vi "Write Register (Core).vi"(0 "SLSC Local in":refnum<class "SLSC Local.lvclass">, 1 "type":enum16{"U8", "U16", "U32", "U64"}(ring), 5 "device":refnum<k21>="$DefaultDevices", 7 "register address":u32 format="%.0x", 9 "data":u64 format="%.0x", 11 "error in (no error)":errorcluster) -> (4 "SLSC Local out":refnum<class "SLSC Local.lvclass">, 6 "device out":refnum<k21>, 8 "next register address":u32 format="%.0x", 15 "error out":errorcluster)   [LabVIEW 2015, in "SLSC Interfaces.lvlib" / "SLSC Local.lvclass"]
uses:
  SLSC Local.lvclass
  <vilib>/SLSC/Write Register (U64).vi
  <vilib>/SLSC/Write Register (U32).vi
  <vilib>/SLSC/Write Register (U16).vi
  <vilib>/SLSC/Write Register (U8).vi
  <vilib>/SLSC/SLSC.lvlib
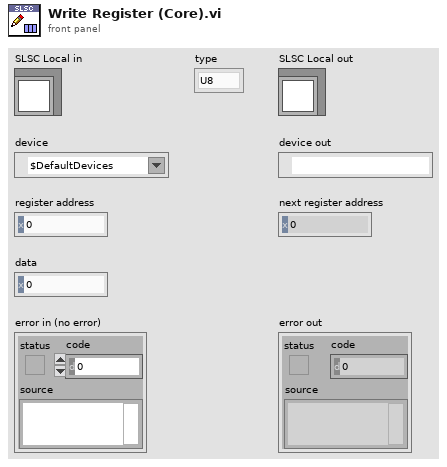
[diagram p1: front panel]
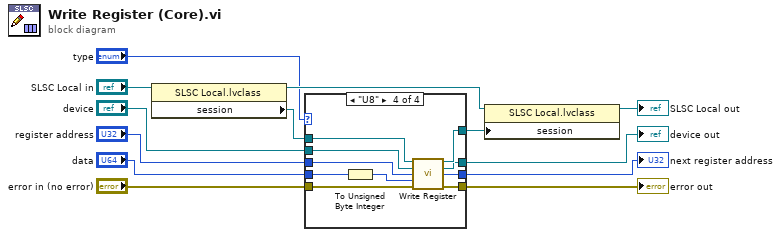
[diagram p0: block diagram]
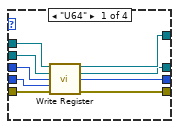
[diagram p2: hidden frame]
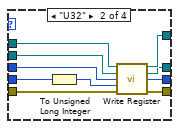
[diagram p3: hidden frame]
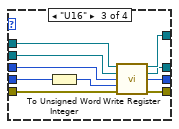
[diagram p4: hidden frame]
diagram:
  n1 = property class="SLSC Local.lvclass"(reference="SLSC Local in") -> (reference out=w6:refnum<class "SLSC Local.lvclass">, "session"=w5:refnum<k21>)  [unwired: 1 in, 1 out]
  n2 = case shown="\"U8\"" "type" {
    tunnel: [w22 w32 w42 w52] -> w13
    tunnel: [w21 w31 w41 w51] -> w12
    tunnel: "error in (no error)" -> [w20 w30 w40 w50]
    tunnel: "data" -> [w19 w24 w34 w44]
    tunnel: "register address" -> [w18 w29 w39 w49]
    tunnel: "device" -> [w17 w28 w38 w48]
    tunnel: w5 -> [w16 w27 w37 w47]
    tunnel: [w15 w26 w36 w46] -> w4
    tunnel: [w14 w25 w35 w45] -> w3
    frame "U64" {
      n3 = call-poly <vilib>:"Write Register.vi"("session in"=w16, "device"=w17, "register address"=w18, "data"=w19, "error in (no error)"=w20) -> ("session out"=w15:refnum<k21>, "device out"=w14:refnum<k21>, "next register address"=w22:u32, "error out"=w21:errorcluster)  [unwired: 7 in]
    }
    frame "U32" {
      n4 = To Unsigned Long Integer(number=w24) -> (unsigned 32bit integer=w23:u32)
      n5 = call-poly <vilib>:"Write Register.vi"("session in"=w27, "device"=w28, "register address"=w29, "data"=w23, "error in (no error)"=w30) -> ("session out"=w26:refnum<k21>, "device out"=w25:refnum<k21>, "next register address"=w32:u32, "error out"=w31:errorcluster)  [unwired: 7 in]
    }
    frame "U16" {
      n6 = To Unsigned Word Integer(number=w34) -> (unsigned 16bit integer=w33:u16)
      n7 = call-poly <vilib>:"Write Register.vi"("session in"=w37, "device"=w38, "register address"=w39, "data"=w33, "error in (no error)"=w40) -> ("session out"=w36:refnum<k21>, "device out"=w35:refnum<k21>, "next register address"=w42:u32, "error out"=w41:errorcluster)  [unwired: 7 in]
    }
    frame "U8" {
      n8 = To Unsigned Byte Integer(number=w44) -> (unsigned 8bit integer=w43:u8)
      n9 = call-poly <vilib>:"Write Register.vi"("session in"=w47, "device"=w48, "register address"=w49, "data"=w43, "error in (no error)"=w50) -> ("session out"=w46:refnum<k21>, "device out"=w45:refnum<k21>, "next register address"=w52:u32, "error out"=w51:errorcluster)  [unwired: 7 in]
    }
  }
  "error out" <- w12
  "device out" <- w3
  "next register address" <- w13
  n10 = property class="SLSC Local.lvclass"(reference=w6, "session"=w4) -> (reference out=→"SLSC Local out":refnum<class "SLSC Local.lvclass">)  [unwired: 1 in, 1 out]
